vi "GetImage.vi"(8 "error in (no error)":errorcluster, 10 "inBufferNumber":u32, 11 "Image Acquisition in":refnum<class "simuCalc.lvclass">) -> (0 "error out":errorcluster, 1 "Cluster":cluster{"processedFPS":dbl, "Buffer Number":u32}, 2 "Image Reference":u16[][](array[numeric]), 3 "Image Acquisition out":refnum<class "simuCalc.lvclass">)   [LabVIEW 2020, in "simuCalc.lvclass"]
uses:
  simuCalc.lvclass
  simuCalc.lvclass/simuCalc.ctl
  <vilib>/numeric/Random Number (Range) DBL.vi
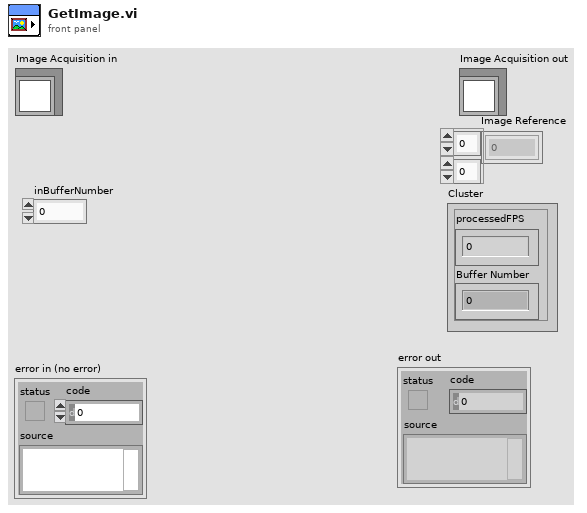
[diagram p1: front panel]
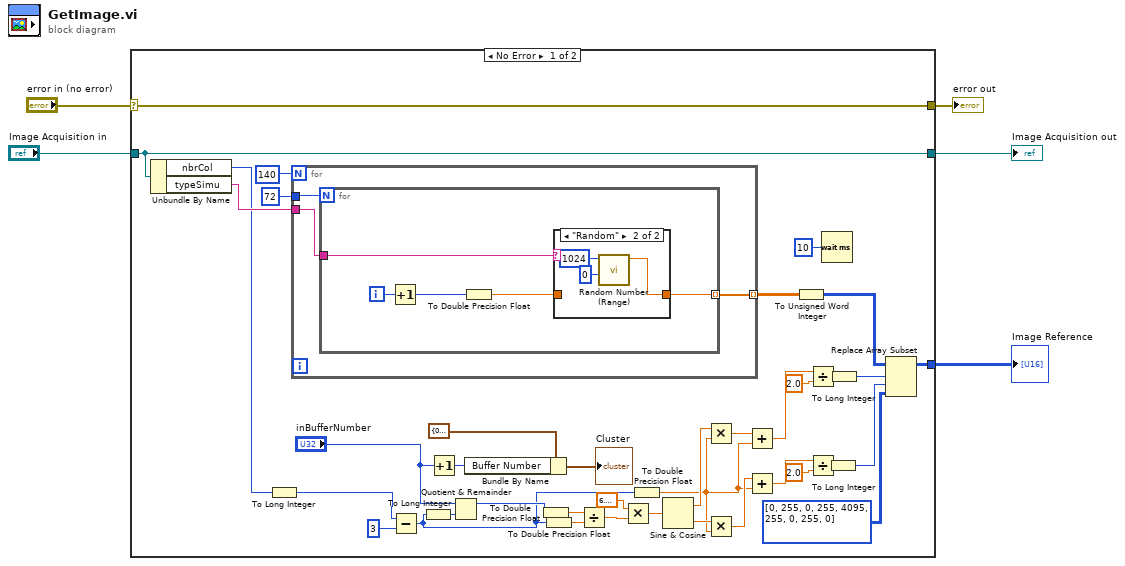
[diagram p0: block diagram]
diagram:
  n1 = case shown="No Error" "error in (no error)" {
    selector: "error in (no error)" -> [w40 w57]
    tunnel: [w40 w57] -> w3
    tunnel: [w35 _] -> w1
    tunnel: [w42 w56] -> w5
    tunnel: "Image Acquisition in" -> [w42 w56]
    frame No Error {
      n2 = Unbundle By Name(w42) -> ("nbrCol"=w16:i32, "typeSimu"=w41:string)
      n3 = To Long Integer(number=w16) -> (32bit integer=w14:i32)
      n4 = for {
        N: 140 -> [_]
        tunnel: [w46] -> w43 mode=indexing
        tunnel: 72 ("nbrCol") -> [w45]
        tunnel: w41 -> [w44]
        n5 = for {
          N: w45 -> [_]
          tunnel: [w51] -> w46 mode=indexing
          tunnel: w44 -> [w50]
          i -> [w48]
          n6 = Increment(x=w48) -> (x+1=w49:i32)
          n7 = To Double Precision Float(number=w49) -> (double precision float=w47:dbl)
          n8 = case shown="\"Random\"" w50 {
            tunnel: [w52 w55] -> w51
            tunnel: w47 -> [w52 _]
            frame "False", Default {
            }
            frame "Random" {
              n9 = call-poly <vilib>:"Random Number (Range).vi"("lower bound (0)"=u64 0, "upper bound (100)"=u64 1024) -> ("number"=w55:dbl)  [unwired: 9 in]
            }
          }
        }
      }
      n10 = Subtract(x=w14, y=3) -> (x-y=w17:i32)
      n11 = To Long Integer(number=w17) -> (32bit integer=w15:i32)
      n12 = Increment(x="inBufferNumber") -> (x+1=w13:u32)
      n13 = Quotient & Remainder(x="inBufferNumber", y=w15) -> (x-y*floor(x/y)=w29:u32)  [unwired: 1 out]
      n14 = Bundle By Name(cluster=cluster{"processedFPS":dbl, "Buffer Number":u32} {"processedFPS"=0.0, "Buffer Number"=0} ("Cluster"), "Buffer Number"=w13) -> (→"Cluster":cluster{"processedFPS":dbl, "Buffer Number":u32})
      n15 = To Double Precision Float(number=w29) -> (double precision float=w12:dbl)
      n16 = To Double Precision Float(number=w17) -> (double precision float=w11:dbl)
      n17 = Divide(x=w12, y=w11) -> (x/y=w27:dbl)
      n18 = Multiply(x=6.283185307179586, y=w27) -> (x*y=w26:dbl)
      n19 = To Double Precision Float(number=w17) -> (double precision float=w10:dbl)
      n20 = Sine & Cosine(0:w26) -> (1:w30:dbl, 2:w31:dbl)
      n21 = Multiply(x=w30, y=w10) -> (x*y=w18:dbl)
      n22 = Multiply(x=w31, y=w10) -> (x*y=w25:dbl)
      n23 = Add(x=w18, y=w10) -> (x+y=w21:dbl)
      n24 = Add(x=w25, y=w10) -> (x+y=w23:dbl)
      n25 = To Unsigned Word Integer(number=w43) -> (unsigned 16bit integer=w36:u16[][])
      n26 = Divide(x=w21, y=2.0) -> (x/y=w19:dbl)
      n27 = Divide(x=w23, y=2.0) -> (x/y=w24:dbl)
      n28 = Wait (ms)(milliseconds to wait=u32 10) -> ()  [unwired: 1 out]
      n29 = To Long Integer(number=w24) -> (32bit integer=w8:i32)
      n30 = To Long Integer(number=w19) -> (32bit integer=w9:i32)
      n31 = Replace Array Subset(array=w36, new element=u16[][] [[0, 255, 0], [255, 4095, 255], [0, 255, 0]], index (row)=w9, index (col)=w8) -> (w35:u16[][])
    }
    frame Error {
    }
  }
  "error out" <- w3
  "Image Acquisition out" <- w5
  "Image Reference" <- w1
